vi "Benchmark Housekeeping.vi"(8 "error in (no error)":errorcluster, 11 "CIFCorePlugin in":refnum<class "CIFCorePlugin.lvclass">) -> (0 "error out":errorcluster, 3 "CIFCorePlugin out":refnum<class "CIFCorePlugin.lvclass">)   [LabVIEW 2021, in "CIFCorePlugin.lvclass"]
uses:
  CIFCorePlugin.lvclass
  CIFCorePlugin.lvclass/CIFCorePlugin.ctl
  <vilib>/CIF Foundation/CIF Utilities/Statistics/I64/Stats_I64_CIF_U.lvclass/Stats_I64_CIF_U.ctl
  Accessors/Timestamps/Read Housekeeping TS.vi
  <vilib>/CIF Foundation/CIF Utilities/Time/System Time/LabVIEW Time to TAI Time.vi
  <vilib>/CIF Foundation/CIF Utilities/Statistics/I64/X1 minus X0.vi/dfabcf33-0dbc-4041-80a5-3dc0c86d2989.vi
  <vilib>/CIF Foundation/CIF Utilities/Statistics/I64/X1 minus X0.vi/dfabcf33-0dbc-4041-80a5-3dc0c86d2989.vi/9eb60a9a-770f-4d2d-8b3f-8465c267ecc9.vi
  <vilib>/CIF Foundation/CIF Utilities/Time/Time_CIF_U.lvlib
  <vilib>/CIF Foundation/CIF Utilities/Statistics/I64/Stats_I64_CIF_U.lvclass
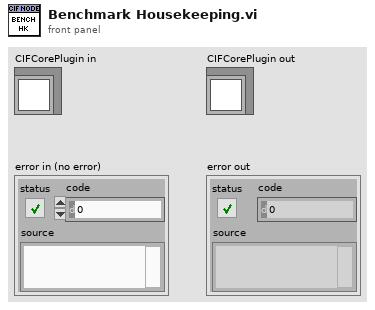
[diagram p1: front panel]
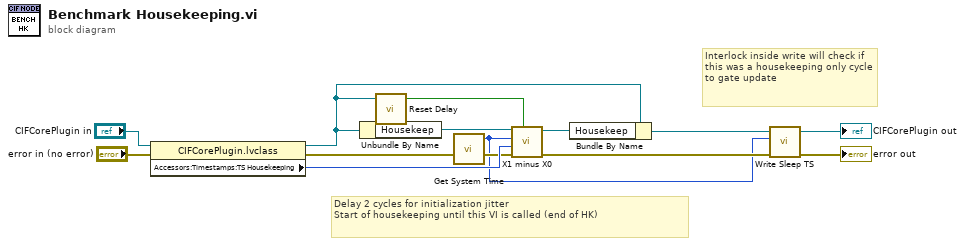
[diagram p0: block diagram]
diagram:
  # "Interlock inside write will check if this was a housekeeping only cycle to gate update"
  # "Delay 2 cycles for initialization jitter\nStart of housekeeping until this VI is called (end of HK)"
  n1 = property class="CIFCorePlugin.lvclass"(reference="CIFCorePlugin in", error in="error in (no error)") -> (reference out=w1:refnum<class "CIFCorePlugin.lvclass">, error out=w7:errorcluster, "Accessors:Timestamps:TS Housekeeping"=w12:i64)
  n2 = Unbundle By Name(w1) -> ("Housekeep"=w11:refnum<class "Stats_I64_CIF_U.lvclass">)
  n3 = call "Reset Delay.vi"("CIFCorePlugin in"=w1) -> ("Reset"=w13:bool)  [unwired: 3 in]
  n4 = call <vilib>:"Get System Time.vi"() -> ("Time (ns)"=w2:i64)  [unwired: 5 in]
  n5 = call <vilib>:"X1 minus X0.vi"("Reinit"=w13, "error in (no error)"=w7, "X0"=w12, "X1"=w2, "Stats_I64_CIF_U in"=w11) -> ("error out"=w5:errorcluster, "Stats_I64_CIF_U out"=w10:refnum<class "Stats_I64_CIF_U.lvclass">)  [unwired: 5 in]
  n6 = Bundle By Name(cluster=w1, "Housekeep"=w10) -> (w6:refnum<class "CIFCorePlugin.lvclass">)
  n7 = call "Write Sleep TS.vi"("error in (no error)"=w5, "Sleep"=w2, "CIFCorePlugin in"=w6) -> ("error out"=→"error out":errorcluster, "CIFCorePlugin out"=→"CIFCorePlugin out":refnum<class "CIFCorePlugin.lvclass">)  [unwired: 7 in]
